vi "Set Channel.vi"(8 "error in (no error)":errorcluster, 10 "Channel Info":T1, 11 "Command Panel in":refnum<class "Command Panel.lvclass">) -> (0 "error out":errorcluster, 3 "Command Panel out":refnum<class "Command Panel.lvclass">)   [LabVIEW 2020, in "VolatusGUI.lvlib" / "Command Panel.lvclass"]
uses:
  Command Panel.lvclass
  Command Panel.lvclass/Command Panel.ctl
  lv-vecto/Vecto/Channel Info.ctl
  lv-vecto/VectoConfig/VectoConfig.lvlib
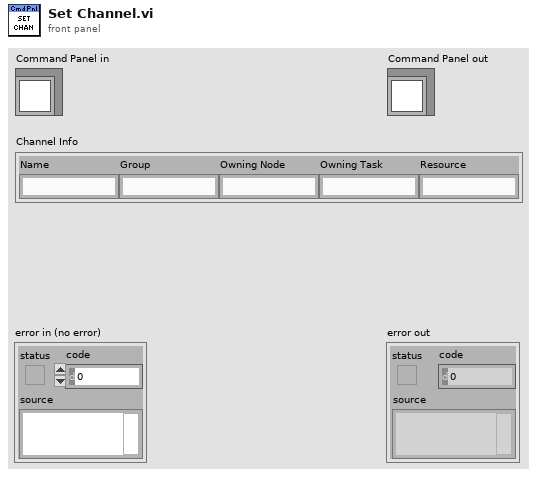
[diagram p1: front panel]
types:
  T1 = typedef "VectoConfig.lvlib/Channel Info.ctl" = cluster{"Name":string, "Group":string, "Owning Node":string, "Owning Task":string, "Resource":string}
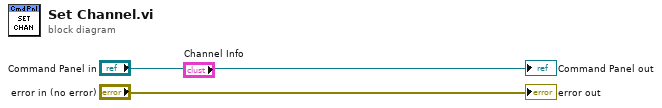
[diagram p0: block diagram]
diagram:
  "error out" <- "error in (no error)"
  "Command Panel out" <- "Command Panel in"
